vi "send_command.vi"(8 "error in (no error)":errorcluster, 10 "GenericCommand.lvclass":refnum<class "GenericCommand.lvclass">, 11 "GenericToplevelComponent in":refnum<class "GenericToplevelComponent.lvclass">) -> (0 "error out":errorcluster, 3 "GenericToplevelComponent out":refnum<class "GenericToplevelComponent.lvclass">, 4 "# elements in queue":i32)   [LabVIEW 2010, in "GenericToplevelComponent.lvclass"]
uses:
  GenericToplevelComponent.lvclass
  components/Command/GenericCommand/GenericCommand/GenericCommand.lvclass
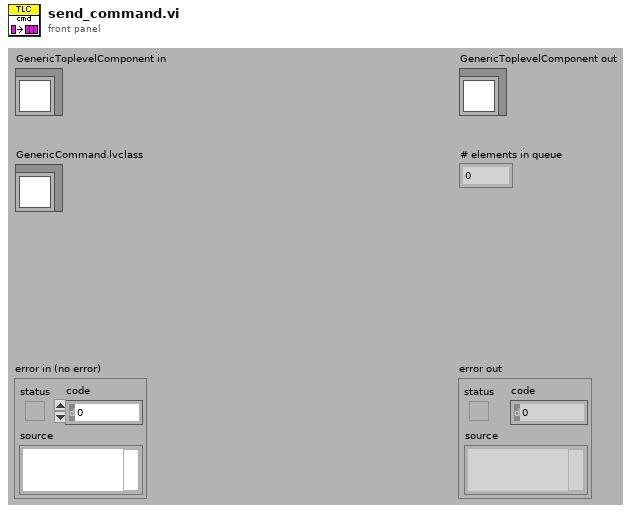
[diagram p1: front panel]
types:
  T1 = typedef "GenericToplevelComponent.lvclass/common_trigger_enum.ctl" = enum16{"NULL", "initialise", "terminate", "fetch command", "fetch data", "attach observer", "register as observer", "detach observer", "acknowledge", "start", "stop", "sweep started", "sweep finished", "experiment started", "experiment stopped"}
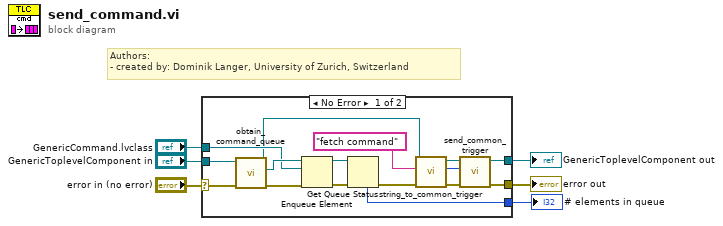
[diagram p0: block diagram]
diagram:
  # "Authors: \n- created by: Dominik Langer, University of Zurich, Switzerland"
  n1 = case shown="No Error" "error in (no error)" {
    selector: "error in (no error)" -> [w20 w24]
    tunnel: [w14 w24] -> w5
    tunnel: [w13 w23] -> w3
    tunnel: "GenericToplevelComponent in" -> [w15 w23]
    tunnel: "GenericCommand.lvclass" -> [w17 _]
    tunnel: [w16 _] -> w1
    frame No Error {
      n2 = call-dynamic "obtain_command_queue.vi"("error in (no error)"=w20, "GenericToplevelComponent in"=w15) -> ("error out"=w22:errorcluster, "command queue"=w19:refnum<queue>, "GenericToplevelComponent out"=w12:refnum<class "GenericToplevelComponent.lvclass">)  [unwired: 7 in]
      n3 = Enqueue Element(queue=w19, element=w17, error in (no error)=w22) -> (queue out=w18:refnum<queue>, error out=w21:errorcluster)  [unwired: 1 in, 1 out]
      n4 = Get Queue Status(queue=w18, error in (no error)=w21) -> (error out=w10:errorcluster, # elements in queue=w16:i32)  [unwired: 1 in, 6 out]
      n5 = call-dynamic "string_to_common_trigger.vi"("error in (no error)"=w10, "trigger string"="fetch command", "GenericToplevelComponent in"=w12) -> ("error out"=w8:errorcluster, "trigger"=w9:T1, "GenericToplevelComponent out"=w11:refnum<class "GenericToplevelComponent.lvclass">)  [unwired: 6 in]
      n6 = call-dynamic "send_common_trigger.vi"("error in (no error)"=w8, "trigger"=w9, "GenericToplevelComponent in"=w11) -> ("error out"=w14:errorcluster, "GenericToplevelComponent out"=w13:refnum<class "GenericToplevelComponent.lvclass">)  [unwired: 6 in, 1 out]
    }
    frame Error {
    }
  }
  "error out" <- w5
  "GenericToplevelComponent out" <- w3
  "# elements in queue" <- w1
